vi "Heater Main.vi"() -> ()   [LabVIEW 2019]
doc: "This example demonstrates how to acquire a continuous amount of data (Waveform) using the DAQ device's internal clock. It also shows how to synchronize two devices for different device families (E Series, S Series, M Series, X Series, DSA, and SC Express), to simultaneously acquire the data.\n\nFor instructions on how to connect your signals to the DAQ device, refer to your device documentation."
uses:
  <vilib>/Utility/error.llb/DialogType.ctl
  <vilib>/DAQmx/write.llb/DAQmx Write (Analog DBL 1Chan 1Samp).vi
  <vilib>/DAQmx/read.llb/DAQmx Read (Analog 1D Wfm NChan NSamp).vi
  <vilib>/DAQmx/configure/timing.llb/DAQmx Timing (Sample Clock).vi
  <vilib>/DAQmx/miscellaneous.llb/DAQmx Fill In Error Info.vi
panel:
  in  "Microhotplate Logger":T1(tab)=enum."Diode"
  in  "Stop":bool
  in  "Enable logging":bool caption="Enable"
  in  "File config":T2={"Filepath"=path "C:/Users/Administrator/Desktop/DAQ Heater Control/Test data", "Test ID"="wo-beam", "PC"="69DTQV2"}
  in  "Sampling config":cluster{"Fs":dbl, "#s":dbl}={"Fs"=1000.0, "#s"=1000.0} {"Fs" format="%.2p"}
  out "Logging":bool
  out "Channel name":string="Diode Voltage"
  in  "Config":T3={"Channel Index"=2, "Diode TC (mV)"=-1.3, "Channel name"="Heater Temperature", "Ref voltage"=0.876, "Ref temp"=25.0, "Gain"=1.0} {"Gain" format="%.3f"; "Ref temp" format="%.3f"; "Ref voltage" format="%.3f"; "Diode TC (mV)" format="%.3f"}
  in  "Config":T3={"Channel Index"=3, "Diode TC (mV)"=-1.3, "Channel name"="Differential Temperature", "Ref voltage"=0.0, "Ref temp"=0.0, "Gain"=1.0} {"Gain" format="%.3f"; "Ref temp" format="%.3f"; "Ref voltage" format="%.3f"; "Diode TC (mV)" format="%.3f"}
  out "Channel name":string="Diode Delta Voltage"
  in  "Heater voltage":dbl=0.8 caption="Amplitude"
  in  "Output channel config":T4={"Output channel"="Dev1/ao0", "name to assign"="Heater Voltage"}
  in  "Heater voltage limit":dbl=2.0 caption="Amplitude"
  in  "INA169 channel config":T5={"Channel Index"=1, "Factor"=0.01, "Channel name"="Heater Current"} {"Factor" format="%.4f"}
  out "INA channel name":string="Heater Shunt"
  in  "IV channel config":T6={"Voltage channel index"=0, "Current channel index"=4}
  out "IV channel names":T7={"Voltage channel name"="Heater Voltage", "Current channel name"="Heater Current"}
  out "Heater delta temperature":dynamicdata(graph)=[{"t0"=timestamp(3663161233.1795554 s since 1904-01-01), "dt"=0.001, "Y"=[0.8018460056446852], "attributes"=variant("NI_ChannelName"=variant(string "Heater Voltage (DC Voltage)"), "NI_OriginalChannelName"=variant(string "Heater Voltage"), "NI_UnitDescription"=variant(string "Volts"))}, {"t0"=timestamp(3663161233.1795664 s since 1904-01-01), "dt"=0.001, "Y"=[0.7325108863741995], "attributes"=variant("NI_ChannelName"=variant(string "Heater Shunt (DC Voltage)"), "NI_OriginalChannelName"=variant(string "Heater Shunt"), "NI_UnitDescription"=variant(string "Volts"))}, {"t0"=timestamp(3663161233.1795774 s since 1904-01-01), "dt"=0.001, "Y"=[0.5244094637105162], "attributes"=variant("NI_ChannelName"=variant(string "Diode Voltage (DC Voltage)"), "NI_OriginalChannelName"=variant(string "Diode Voltage"), "NI_UnitDescription"=variant(string "Volts"))}, {"t0"=timestamp(3663161233.1795883 s since 1904-01-01), "dt"=0.001, "Y"=[-0.02927033778076672], "attributes"=variant("NI_ChannelName"=variant(string "Diode Delta Voltage (DC Voltage)"), "NI_OriginalChannelName"=variant(string "Diode Delta Voltage"), "NI_UnitDescription"=variant(string "Volts"))}, {"t0"=timestamp(3663161233.1795554 s since 1904-01-01), "dt"=0.001, "Y"=[0.005873609285933641], "attributes"=variant("NI_ChannelName"=variant(string "Heater Resistance (DC Voltage)"), "NI_OriginalChannelName"=variant(string "Heater Resistance"), "NI_UnitDescription"=variant(string "Ohms"))}, {"t0"=timestamp(3663161233.1795554 s since 1904-01-01), "dt"=0.001, "Y"=[0.005873609285933641], "attributes"=variant("NI_ChannelName"=variant(string "Heater Resistance (DC Voltage)"), "NI_OriginalChannelName"=variant(string "Heater Resistance"), "NI_UnitDescription"=variant(string "Ohms"))}, {"t0"=timestamp(3663161233.1795774 s since 1904-01-01), "dt"=0.001, "Y"=[295.4542586842174], "attributes"=variant("NI_ChannelName"=variant(string "Heater Temperature (DC Voltage)"), "NI_OriginalChannelName"=variant(string "Heater Temperature"), "NI_UnitDescription"=variant(string "degC"))}, {"t0"=timestamp(3663161233.1795883 s since 1904-01-01), "dt"=0.001, "Y"=[47.5156444467435], "attributes"=variant("NI_ChannelName"=variant(string "Differential Temperature (DC Voltage)"), "NI_OriginalChannelName"=variant(string "Differential Temperature"), "NI_UnitDescription"=variant(string "degC"))}]
  out "Diode voltage - differential":dynamicdata(graph)=[{"t0"=timestamp(3663161233.1795554 s since 1904-01-01), "dt"=0.001, "Y"=[0.8018460056446852], "attributes"=variant("NI_ChannelName"=variant(string "Heater Voltage (DC Voltage)"), "NI_OriginalChannelName"=variant(string "Heater Voltage"), "NI_UnitDescription"=variant(string "Volts"))}, {"t0"=timestamp(3663161233.1795664 s since 1904-01-01), "dt"=0.001, "Y"=[0.7325108863741995], "attributes"=variant("NI_ChannelName"=variant(string "Heater Shunt (DC Voltage)"), "NI_OriginalChannelName"=variant(string "Heater Shunt"), "NI_UnitDescription"=variant(string "Volts"))}, {"t0"=timestamp(3663161233.1795774 s since 1904-01-01), "dt"=0.001, "Y"=[0.5244094637105162], "attributes"=variant("NI_ChannelName"=variant(string "Diode Voltage (DC Voltage)"), "NI_OriginalChannelName"=variant(string "Diode Voltage"), "NI_UnitDescription"=variant(string "Volts"))}, {"t0"=timestamp(3663161233.1795883 s since 1904-01-01), "dt"=0.001, "Y"=[-0.02927033778076672], "attributes"=variant("NI_ChannelName"=variant(string "Diode Delta Voltage (DC Voltage)"), "NI_OriginalChannelName"=variant(string "Diode Delta Voltage"), "NI_UnitDescription"=variant(string "Volts"))}, {"t0"=timestamp(3663161233.1795554 s since 1904-01-01), "dt"=0.001, "Y"=[0.005873609285933641], "attributes"=variant("NI_ChannelName"=variant(string "Heater Resistance (DC Voltage)"), "NI_OriginalChannelName"=variant(string "Heater Resistance"), "NI_UnitDescription"=variant(string "Ohms"))}, {"t0"=timestamp(3663161233.1795554 s since 1904-01-01), "dt"=0.001, "Y"=[0.005873609285933641], "attributes"=variant("NI_ChannelName"=variant(string "Heater Resistance (DC Voltage)"), "NI_OriginalChannelName"=variant(string "Heater Resistance"), "NI_UnitDescription"=variant(string "Ohms"))}, {"t0"=timestamp(3663161233.1795774 s since 1904-01-01), "dt"=0.001, "Y"=[295.4542586842174], "attributes"=variant("NI_ChannelName"=variant(string "Heater Temperature (DC Voltage)"), "NI_OriginalChannelName"=variant(string "Heater Temperature"), "NI_UnitDescription"=variant(string "degC"))}, {"t0"=timestamp(3663161233.1795883 s since 1904-01-01), "dt"=0.001, "Y"=[47.5156444467435], "attributes"=variant("NI_ChannelName"=variant(string "Differential Temperature (DC Voltage)"), "NI_OriginalChannelName"=variant(string "Differential Temperature"), "NI_UnitDescription"=variant(string "degC"))}]
  out "Heater temperature - Diode":dynamicdata(graph)=[{"t0"=timestamp(3663161233.1795554 s since 1904-01-01), "dt"=0.001, "Y"=[0.8018460056446852], "attributes"=variant("NI_ChannelName"=variant(string "Heater Voltage (DC Voltage)"), "NI_OriginalChannelName"=variant(string "Heater Voltage"), "NI_UnitDescription"=variant(string "Volts"))}, {"t0"=timestamp(3663161233.1795664 s since 1904-01-01), "dt"=0.001, "Y"=[0.7325108863741995], "attributes"=variant("NI_ChannelName"=variant(string "Heater Shunt (DC Voltage)"), "NI_OriginalChannelName"=variant(string "Heater Shunt"), "NI_UnitDescription"=variant(string "Volts"))}, {"t0"=timestamp(3663161233.1795774 s since 1904-01-01), "dt"=0.001, "Y"=[0.5244094637105162], "attributes"=variant("NI_ChannelName"=variant(string "Diode Voltage (DC Voltage)"), "NI_OriginalChannelName"=variant(string "Diode Voltage"), "NI_UnitDescription"=variant(string "Volts"))}, {"t0"=timestamp(3663161233.1795883 s since 1904-01-01), "dt"=0.001, "Y"=[-0.02927033778076672], "attributes"=variant("NI_ChannelName"=variant(string "Diode Delta Voltage (DC Voltage)"), "NI_OriginalChannelName"=variant(string "Diode Delta Voltage"), "NI_UnitDescription"=variant(string "Volts"))}, {"t0"=timestamp(3663161233.1795554 s since 1904-01-01), "dt"=0.001, "Y"=[0.005873609285933641], "attributes"=variant("NI_ChannelName"=variant(string "Heater Resistance (DC Voltage)"), "NI_OriginalChannelName"=variant(string "Heater Resistance"), "NI_UnitDescription"=variant(string "Ohms"))}, {"t0"=timestamp(3663161233.1795554 s since 1904-01-01), "dt"=0.001, "Y"=[0.005873609285933641], "attributes"=variant("NI_ChannelName"=variant(string "Heater Resistance (DC Voltage)"), "NI_OriginalChannelName"=variant(string "Heater Resistance"), "NI_UnitDescription"=variant(string "Ohms"))}, {"t0"=timestamp(3663161233.1795774 s since 1904-01-01), "dt"=0.001, "Y"=[295.4542586842174], "attributes"=variant("NI_ChannelName"=variant(string "Heater Temperature (DC Voltage)"), "NI_OriginalChannelName"=variant(string "Heater Temperature"), "NI_UnitDescription"=variant(string "degC"))}, {"t0"=timestamp(3663161233.1795883 s since 1904-01-01), "dt"=0.001, "Y"=[47.5156444467435], "attributes"=variant("NI_ChannelName"=variant(string "Differential Temperature (DC Voltage)"), "NI_OriginalChannelName"=variant(string "Differential Temperature"), "NI_UnitDescription"=variant(string "degC"))}]
  out "Heater current":dynamicdata(graph)=[{"t0"=timestamp(3663161233.1795554 s since 1904-01-01), "dt"=0.001, "Y"=[0.8018460056446852], "attributes"=variant("NI_ChannelName"=variant(string "Heater Voltage (DC Voltage)"), "NI_OriginalChannelName"=variant(string "Heater Voltage"), "NI_UnitDescription"=variant(string "Volts"))}, {"t0"=timestamp(3663161233.1795664 s since 1904-01-01), "dt"=0.001, "Y"=[0.7325108863741995], "attributes"=variant("NI_ChannelName"=variant(string "Heater Shunt (DC Voltage)"), "NI_OriginalChannelName"=variant(string "Heater Shunt"), "NI_UnitDescription"=variant(string "Volts"))}, {"t0"=timestamp(3663161233.1795774 s since 1904-01-01), "dt"=0.001, "Y"=[0.5244094637105162], "attributes"=variant("NI_ChannelName"=variant(string "Diode Voltage (DC Voltage)"), "NI_OriginalChannelName"=variant(string "Diode Voltage"), "NI_UnitDescription"=variant(string "Volts"))}, {"t0"=timestamp(3663161233.1795883 s since 1904-01-01), "dt"=0.001, "Y"=[-0.02927033778076672], "attributes"=variant("NI_ChannelName"=variant(string "Diode Delta Voltage (DC Voltage)"), "NI_OriginalChannelName"=variant(string "Diode Delta Voltage"), "NI_UnitDescription"=variant(string "Volts"))}, {"t0"=timestamp(3663161233.1795554 s since 1904-01-01), "dt"=0.001, "Y"=[0.005873609285933641], "attributes"=variant("NI_ChannelName"=variant(string "Heater Resistance (DC Voltage)"), "NI_OriginalChannelName"=variant(string "Heater Resistance"), "NI_UnitDescription"=variant(string "Ohms"))}, {"t0"=timestamp(3663161233.1795554 s since 1904-01-01), "dt"=0.001, "Y"=[0.005873609285933641], "attributes"=variant("NI_ChannelName"=variant(string "Heater Resistance (DC Voltage)"), "NI_OriginalChannelName"=variant(string "Heater Resistance"), "NI_UnitDescription"=variant(string "Ohms"))}, {"t0"=timestamp(3663161233.1795774 s since 1904-01-01), "dt"=0.001, "Y"=[295.4542586842174], "attributes"=variant("NI_ChannelName"=variant(string "Heater Temperature (DC Voltage)"), "NI_OriginalChannelName"=variant(string "Heater Temperature"), "NI_UnitDescription"=variant(string "degC"))}, {"t0"=timestamp(3663161233.1795883 s since 1904-01-01), "dt"=0.001, "Y"=[47.5156444467435], "attributes"=variant("NI_ChannelName"=variant(string "Differential Temperature (DC Voltage)"), "NI_OriginalChannelName"=variant(string "Differential Temperature"), "NI_UnitDescription"=variant(string "degC"))}]
  out "Heater voltage":dynamicdata(graph)=[{"t0"=timestamp(3663161233.1795554 s since 1904-01-01), "dt"=0.001, "Y"=[0.8018460056446852], "attributes"=variant("NI_ChannelName"=variant(string "Heater Voltage (DC Voltage)"), "NI_OriginalChannelName"=variant(string "Heater Voltage"), "NI_UnitDescription"=variant(string "Volts"))}, {"t0"=timestamp(3663161233.1795664 s since 1904-01-01), "dt"=0.001, "Y"=[0.7325108863741995], "attributes"=variant("NI_ChannelName"=variant(string "Heater Shunt (DC Voltage)"), "NI_OriginalChannelName"=variant(string "Heater Shunt"), "NI_UnitDescription"=variant(string "Volts"))}, {"t0"=timestamp(3663161233.1795774 s since 1904-01-01), "dt"=0.001, "Y"=[0.5244094637105162], "attributes"=variant("NI_ChannelName"=variant(string "Diode Voltage (DC Voltage)"), "NI_OriginalChannelName"=variant(string "Diode Voltage"), "NI_UnitDescription"=variant(string "Volts"))}, {"t0"=timestamp(3663161233.1795883 s since 1904-01-01), "dt"=0.001, "Y"=[-0.02927033778076672], "attributes"=variant("NI_ChannelName"=variant(string "Diode Delta Voltage (DC Voltage)"), "NI_OriginalChannelName"=variant(string "Diode Delta Voltage"), "NI_UnitDescription"=variant(string "Volts"))}, {"t0"=timestamp(3663161233.1795554 s since 1904-01-01), "dt"=0.001, "Y"=[0.005873609285933641], "attributes"=variant("NI_ChannelName"=variant(string "Heater Resistance (DC Voltage)"), "NI_OriginalChannelName"=variant(string "Heater Resistance"), "NI_UnitDescription"=variant(string "Ohms"))}, {"t0"=timestamp(3663161233.1795554 s since 1904-01-01), "dt"=0.001, "Y"=[0.005873609285933641], "attributes"=variant("NI_ChannelName"=variant(string "Heater Resistance (DC Voltage)"), "NI_OriginalChannelName"=variant(string "Heater Resistance"), "NI_UnitDescription"=variant(string "Ohms"))}, {"t0"=timestamp(3663161233.1795774 s since 1904-01-01), "dt"=0.001, "Y"=[295.4542586842174], "attributes"=variant("NI_ChannelName"=variant(string "Heater Temperature (DC Voltage)"), "NI_OriginalChannelName"=variant(string "Heater Temperature"), "NI_UnitDescription"=variant(string "degC"))}, {"t0"=timestamp(3663161233.1795883 s since 1904-01-01), "dt"=0.001, "Y"=[47.5156444467435], "attributes"=variant("NI_ChannelName"=variant(string "Differential Temperature (DC Voltage)"), "NI_OriginalChannelName"=variant(string "Differential Temperature"), "NI_UnitDescription"=variant(string "degC"))}]
  out "Diode voltage":dynamicdata(graph)=[{"t0"=timestamp(3663161233.1795554 s since 1904-01-01), "dt"=0.001, "Y"=[0.8018460056446852], "attributes"=variant("NI_ChannelName"=variant(string "Heater Voltage (DC Voltage)"), "NI_OriginalChannelName"=variant(string "Heater Voltage"), "NI_UnitDescription"=variant(string "Volts"))}, {"t0"=timestamp(3663161233.1795664 s since 1904-01-01), "dt"=0.001, "Y"=[0.7325108863741995], "attributes"=variant("NI_ChannelName"=variant(string "Heater Shunt (DC Voltage)"), "NI_OriginalChannelName"=variant(string "Heater Shunt"), "NI_UnitDescription"=variant(string "Volts"))}, {"t0"=timestamp(3663161233.1795774 s since 1904-01-01), "dt"=0.001, "Y"=[0.5244094637105162], "attributes"=variant("NI_ChannelName"=variant(string "Diode Voltage (DC Voltage)"), "NI_OriginalChannelName"=variant(string "Diode Voltage"), "NI_UnitDescription"=variant(string "Volts"))}, {"t0"=timestamp(3663161233.1795883 s since 1904-01-01), "dt"=0.001, "Y"=[-0.02927033778076672], "attributes"=variant("NI_ChannelName"=variant(string "Diode Delta Voltage (DC Voltage)"), "NI_OriginalChannelName"=variant(string "Diode Delta Voltage"), "NI_UnitDescription"=variant(string "Volts"))}, {"t0"=timestamp(3663161233.1795554 s since 1904-01-01), "dt"=0.001, "Y"=[0.005873609285933641], "attributes"=variant("NI_ChannelName"=variant(string "Heater Resistance (DC Voltage)"), "NI_OriginalChannelName"=variant(string "Heater Resistance"), "NI_UnitDescription"=variant(string "Ohms"))}, {"t0"=timestamp(3663161233.1795554 s since 1904-01-01), "dt"=0.001, "Y"=[0.005873609285933641], "attributes"=variant("NI_ChannelName"=variant(string "Heater Resistance (DC Voltage)"), "NI_OriginalChannelName"=variant(string "Heater Resistance"), "NI_UnitDescription"=variant(string "Ohms"))}, {"t0"=timestamp(3663161233.1795774 s since 1904-01-01), "dt"=0.001, "Y"=[295.4542586842174], "attributes"=variant("NI_ChannelName"=variant(string "Heater Temperature (DC Voltage)"), "NI_OriginalChannelName"=variant(string "Heater Temperature"), "NI_UnitDescription"=variant(string "degC"))}, {"t0"=timestamp(3663161233.1795883 s since 1904-01-01), "dt"=0.001, "Y"=[47.5156444467435], "attributes"=variant("NI_ChannelName"=variant(string "Differential Temperature (DC Voltage)"), "NI_OriginalChannelName"=variant(string "Differential Temperature"), "NI_UnitDescription"=variant(string "degC"))}]
  in  "Channel 4 config":T8={"Channel"="Dev1/ai1", "Vmax"=1.0, "Vmin"=0.0, "name to assign"="Diode Delta Voltage", "input terminal configuration"=10083} {"input terminal configuration" items=["Default"=-1, "RSE"=10083, "NRSE"=10078, "Differential"=10106, "Pseudodifferential"=12529]; "Vmin" format="%0.2f"; "Vmax" format="%0.2f"}
  in  "Channel 2 config":T8={"Channel"="Dev1/ai3", "Vmax"=1.0, "Vmin"=0.0, "name to assign"="Heater Shunt", "input terminal configuration"=10083} {"input terminal configuration" items=["Default"=-1, "RSE"=10083, "NRSE"=10078, "Differential"=10106, "Pseudodifferential"=12529]; "Vmin" format="%0.2f"; "Vmax" format="%0.2f"}
  in  "Channel 1 config":T8={"Channel"="Dev1/ai2", "Vmax"=2.0, "Vmin"=0.0, "name to assign"="Heater Voltage", "input terminal configuration"=10106} {"input terminal configuration" items=["Default"=-1, "RSE"=10083, "NRSE"=10078, "Differential"=10106, "Pseudodifferential"=12529]; "Vmin" format="%0.2f"; "Vmax" format="%0.2f"}
  in  "Channel 3 config":T8={"Channel"="Dev1/ai4", "Vmax"=1.0, "Vmin"=0.0, "name to assign"="Diode Voltage", "input terminal configuration"=10083} {"input terminal configuration" items=["Default"=-1, "RSE"=10083, "NRSE"=10078, "Differential"=10106, "Pseudodifferential"=12529]; "Vmin" format="%0.2f"; "Vmax" format="%0.2f"}
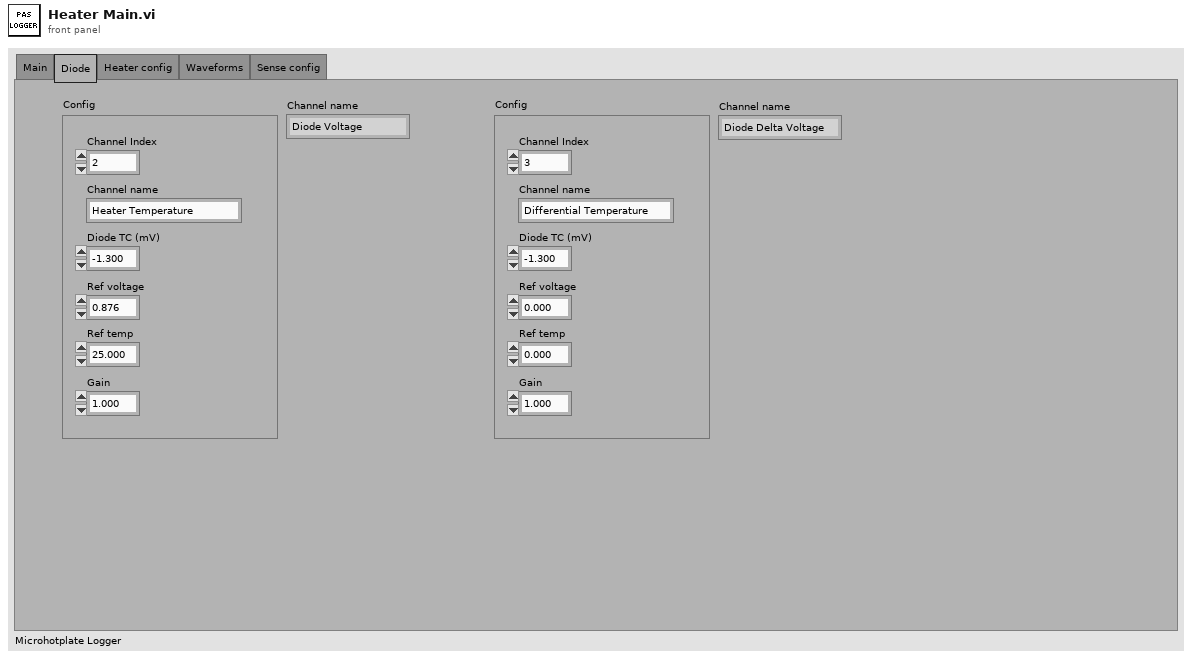
[diagram p1: front panel]
types:
  T1 = enum32{"Main", "Diode", "Heater config", "Waveforms", "Sense config"}
  T2 = cluster{"Filepath":path, "Test ID":string, "PC":string}
  T3 = cluster{"Channel Index":i32, "Diode TC (mV)":dbl, "Channel name":string, "Ref voltage":dbl, "Ref temp":dbl, "Gain":dbl}
  T4 = cluster{"Output channel":tag, "name to assign":string}
  T5 = cluster{"Channel Index":i32, "Factor":dbl, "Channel name":string}
  T6 = cluster{"Voltage channel index":i32, "Current channel index":i32}
  T7 = cluster{"Voltage channel name":string, "Current channel name":string}
  T8 = cluster{"Channel":tag, "Vmax":dbl, "Vmin":dbl, "name to assign":string, "input terminal configuration":i32}
  T9 = typedef "DialogType.ctl" = u16
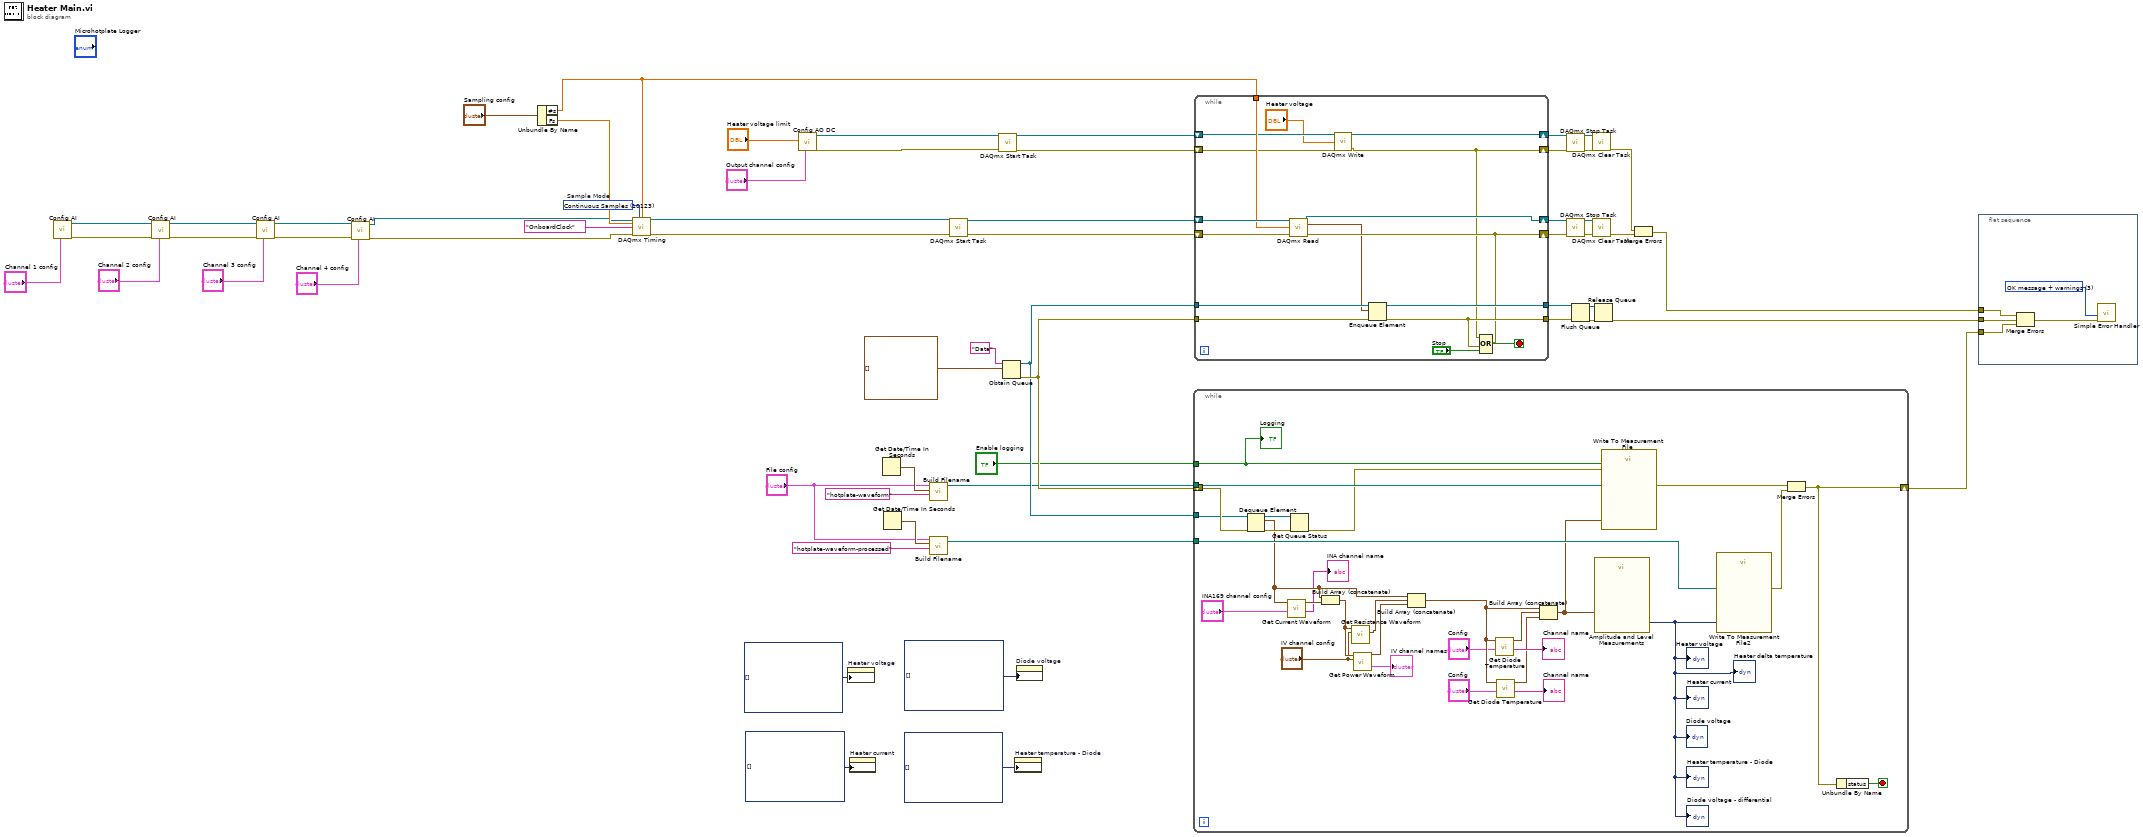
[diagram p0: block diagram]
diagram:
  w50 = 10123 items=["Finite Samples"=10178, "Continuous Samples"=10123, "Hardware Timed Single Point"=12522]  # Sample Mode
  n1 = call "Config AI.vi"("Channel config"="Channel 1 config") -> ("error out"=w29:errorcluster, "task out"=w28:refnum<k21>)  [unwired: 9 in]
  n2 = call "Config AI.vi"("Channel config"="Channel 2 config", "error in"=w29, "task in"=w28) -> ("error out"=w19:errorcluster, "task out"=w18:refnum<k21>)  [unwired: 7 in]
  n3 = call "Config AI.vi"("Channel config"="Channel 3 config", "error in"=w19, "task in"=w18) -> ("error out"=w14:errorcluster, "task out"=w13:refnum<k21>)  [unwired: 7 in]
  n4 = call "Config AI.vi"("Channel config"="Channel 4 config", "error in"=w14, "task in"=w13) -> ("error out"=w11:errorcluster, "task out"=w12:refnum<k21>)  [unwired: 7 in]
  n5 = Unbundle By Name("Sampling config") -> ("#s"=w31:dbl, "Fs"=w30:dbl)
  n6 = call-poly <vilib>:"DAQmx Timing.vi"("task/channels in"=w12, "sample mode"=w50, "samples per channel"=w31, "rate"=w30, "source"=tag "OnboardClock", "error in"=w11) -> ("task out"=w6:refnum<k21>, "error out"=w5:errorcluster)  [unwired: 8 in]
  n7 = call "Config AO DC.vi"("Channel config"="Output channel config", "Voltage"="Heater voltage limit") -> ("error out"=w44:errorcluster, "task out"=w45:refnum<k21>)  [unwired: 8 in]
  n8 = property on="Heater voltage" class="WFChart (strict)"("History Data"=dynamicdata[] []) -> ()  [unwired: 2 in, 2 out]
  n9 = property on="Heater current" class="WFChart (strict)"("History Data"=dynamicdata[] []) -> ()  [unwired: 2 in, 2 out]
  n10 = Get Date/Time In Seconds() -> (seconds since 1Jan1904=w22:timestamp)
  n11 = Get Date/Time In Seconds() -> (seconds since 1Jan1904=w9:timestamp)
  n12 = call "Build Filename.vi"("Test type"="hotplate-waveform" ("File type"), "time stamp"=w22, "File config"="File config") -> ("appended path"=w24:path)  [unwired: 8 in]
  n13 = call "Build Filename.vi"("Test type"="hotplate-waveform-processed" ("File type"), "time stamp"=w9, "File config"="File config") -> ("appended path"=w8:path)  [unwired: 8 in]
  n14 = call <vilib>:"DAQmx Start Task.vi"("task/channels in"=w6, "error in"=w5) -> ("task out"=w46:refnum<k21>, "error out"=w47:errorcluster)  [unwired: 12 in]
  n15 = call <vilib>:"DAQmx Start Task.vi"("task/channels in"=w45, "error in"=w44) -> ("task out"=w48:refnum<k21>, "error out"=w49:errorcluster)  [unwired: 12 in]
  n16 = Obtain Queue(name (unnamed)="Data" ("名前（名前なし）"), element data type=waveform(dbl)[] [] ("data")) -> (queue out=w34:refnum<queue>, error out=w35:errorcluster)  [unwired: 3 in, 1 out]
  n17 = property on="Heater temperature - Diode" class="WFChart (strict)"("History Data"=dynamicdata[] []) -> ()  [unwired: 2 in, 2 out]
  n18 = property on="Diode voltage" class="WFChart (strict)"("History Data"=dynamicdata[] []) -> ()  [unwired: 2 in, 2 out]
  n19 = while {
    tunnel: w34 -> [w89]
    shift-right: [w82] -> w33
    shift-left: w35 -> [w90]
    tunnel: w24 -> [w88]
    tunnel: "Enable logging" -> [w84]
    tunnel: w8 -> [w78]
    stop <- w81 stop-if-true
    n20 = Dequeue Element(queue=w89, error in (no error)=w90) -> (queue out=w86:refnum<queue>, element=w72:waveform(dbl)[], error out=w87:errorcluster)  [unwired: 1 in, 1 out]
    n21 = call "Get Current Waveform.vi"("Config"="INA169 channel config", "array"=w72) -> ("Channel name"=→"INA channel name":string, "Current waveform out"=w75:waveform(dbl))  [unwired: 8 in]
    n22 = Get Queue Status(queue=w86, error in (no error)=w87) -> (error out=w85:errorcluster)  [unwired: 1 in, 7 out]
    n23 = Build Array (concatenate)(w72, w75) -> (w63:waveform(dbl)[])
    n24 = call "Get Resistance Waveform.vi"("Channel config"="IV channel config", "array"=w63) -> ("Resistance waveform out"=w61:waveform(dbl))  [unwired: 8 in, 1 out]
    n25 = call "Get Power Waveform.vi"("Channel config"="IV channel config", "array"=w63) -> ("Power waveform out"=w74:waveform(dbl), "Channel names"=→"IV channel names":T7)  [unwired: 8 in]
    n26 = Build Array (concatenate)(w72, w61, w74) -> (w69:waveform(dbl)[])
    n27 = call "Get Diode Temperature.vi"("Config"="Config", "array"=w69) -> ("Channel name"=→"Channel name":string, "waveform out"=w66:waveform(dbl))  [unwired: 8 in]
    n28 = call "Get Diode Temperature.vi"("Config"="Config", "array"=w69) -> ("Channel name"=→"Channel name":string, "waveform out"=w65:waveform(dbl))  [unwired: 8 in]
    n29 = Build Array (concatenate)(w69, w66, w65) -> (w77:waveform(dbl)[])
    n30 = call "Amplitude and Level Measurements"("Signals"=w77) -> ("Mean (DC)"=w64:dynamicdata)  [unwired: 13 in, 1 out]
    "Heater voltage" <- w64
    "Heater current" <- w64
    "Diode voltage" <- w64
    "Heater temperature - Diode" <- w64
    "Diode voltage - differential" <- w64
    "Heater delta temperature" <- w64
    n31 = call "Write To Measurement File"("Signals"=w77, "Enable"=w84, "error in (no error)"=w85, "Filename"=w88) -> ("error out"=w83:errorcluster)  [unwired: 13 in, 2 out]
    n32 = call "Write To Measurement File2"("Signals"=w64, "Filename"=w78) -> ("error out"=w79:errorcluster)  [unwired: 15 in, 2 out]
    n33 = Merge Errors(w83, w79) -> (w82:errorcluster)
    n34 = Unbundle By Name(w82) -> ("status"=w81:bool)
    "Logging" <- w84
  }
  n35 = while {
    shift-right: [w94] -> w59
    shift-left: w49 -> [w95]
    shift-right: [w97] -> w55
    shift-left: w47 -> [w105]
    shift-right: [w92] -> w60
    shift-left: w48 -> [w93]
    shift-right: [w104] -> w56
    shift-left: w46 -> [w106]
    tunnel: w31 -> [w103]
    tunnel: [w102] -> w40
    tunnel: [w98] -> w39
    tunnel: w34 -> [w101]
    tunnel: w35 -> [w100]
    stop <- w107 stop-if-true
    n36 = call-poly <vilib>:"DAQmx Read.vi"("task/channels in"=w106, "number of samples per channel"=w103, "error in"=w105) -> ("task out"=w104:refnum<k21>, "data"=w96:waveform(dbl)[], "error out"=w97:errorcluster)  [unwired: 10 in]
    n37 = call-poly <vilib>:"DAQmx Write.vi"("task/channels in"=w93, "data"="Heater voltage", "error in"=w95) -> ("task out"=w92:refnum<k21>, "error out"=w94:errorcluster)  [unwired: 10 in, 1 out]
    n38 = Enqueue Element(queue=w101, element=w96, error in (no error)=w100) -> (queue out=w102:refnum<queue>, error out=w98:errorcluster)  [unwired: 1 in, 1 out]
    n39 = Compound Arithmetic op=OR(w94, w97, w98, "Stop") -> (w107:bool)
  }
  n40 = call <vilib>:"DAQmx Stop Task.vi"("task/channels in"=w60, "error in"=w59) -> ("task out"=w57:refnum<k21>, "error out"=w58:errorcluster)  [unwired: 12 in]
  n41 = call <vilib>:"DAQmx Stop Task.vi"("task/channels in"=w56, "error in"=w55) -> ("task out"=w53:refnum<k21>, "error out"=w54:errorcluster)  [unwired: 12 in]
  n42 = Flush Queue(queue=w40, error in (no error)=w39) -> (queue out=w41:refnum<queue>, error out=w42:errorcluster)  [unwired: 1 out]
  n43 = call <vilib>:"DAQmx Clear Task.vi"("task in"=w57, "error in"=w58) -> ("error out"=w52:errorcluster)  [unwired: 13 in]
  n44 = call <vilib>:"DAQmx Clear Task.vi"("task in"=w53, "error in"=w54) -> ("error out"=w51:errorcluster)  [unwired: 13 in]
  n45 = Release Queue(queue=w41, error in (no error)=w42) -> (error out=w37:errorcluster)  [unwired: 1 in, 2 out]
  n46 = Merge Errors(w52, w51) -> (w38:errorcluster)
  n47 = flat-sequence {
    tunnel: w38 -> [w112]
    tunnel: w37 -> [w111]
    tunnel: w33 -> [w108]
    frame #0 {
      w110 = T9 3 items=["no dialog", "OK message", "continue or stop message", "OK message + warnings", "continue/stop + warnings"] ("type of dialog (OK msg:1)")
      n48 = Merge Errors(w112, w111, w108) -> (w109:errorcluster)
      n49 = call <vilib>:"Simple Error Handler.vi"("type of dialog (OK msg:1)"=w110, "error in (no error)"=w109) -> ()  [unwired: 3 in, 5 out]
    }
  }
